vi "AtSpectrograph_cancelCallback_logEvent_STRING.vi"(8 "error in (no error)":errorcluster) -> (0 "error out":errorcluster, 3 "function return":i32)   [LabVIEW 2016, in "SALLV_AtSpectrograph.lvlib"]
doc: "int AtSpectrograph_shm_cancelCallback_logevent_STRINGLV();"
uses:
  SALLV_AtSpectrograph.lvlib
  SALLV_AtSpectrograph.so
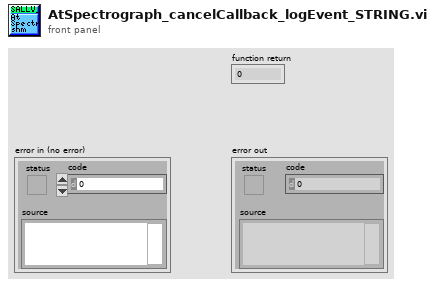
[diagram p1: front panel]
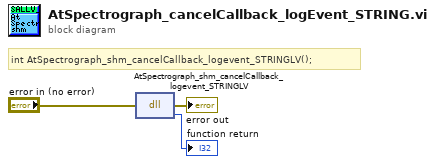
[diagram p0: block diagram]
diagram:
  # "int AtSpectrograph_shm_cancelCallback_logevent_STRINGLV();"
  n1 = dll-call lib="home/harini/tcs/temp/SALLV_AtSpectrograph/SALLV_AtSpectrograph.*" fn="AtSpectrograph_shm_cancelCallback_logevent_STRINGLV"(error in="error in (no error)") -> (error out=→"error out":errorcluster, →"function return":i32)  [unwired: 2 in, 1 out]
